vi "stimulate_and_record_async_daq_temp.vi"(3 "SSH password":string, 4 "Transfer and Run Date Folder After Experiment":bool, 5 "SSH user name":string, 6 "Tags":string, 7 "Frames":i32, 8 "Convert Power to Voltage":bool, 9 "voltages/power":dbl[](array[numeric]), 10 "parameters":string[](array[string]), 11 "parameters headers":string[](array[string])) -> ()   [LabVIEW 2016]
uses:
  <vilib>/vision/driver/IMAQdx.llb/IMAQdx Acquisition Mode.ctl
  <vilib>/userdefined/High Color/IMAQdx.ctl
  <vilib>/vision/driver/IMAQdx.llb/IMAQdx Buffer Number Mode.ctl
  <vilib>/Utility/file.llb/Write To Spreadsheet File (DBL).vi
  <vilib>/Utility/file.llb/Write To Spreadsheet File (string).vi
  <vilib>/Utility/file.llb/Read From Spreadsheet File (string).vi
  <vilib>/vision/driver/NI_Vision_Acquisition_Software.lvlib
panel:
  out "DAC0 Voltage":dbl format="%.6f"
  out "Saved Buffer Number":u32
  out "ProcessFrameRate":dbl
  out "# elements in queue":i32
  out "CameraFrameRate":dbl
  out "Camera Buffer Number":u32
  out "Image":T1(plugin-control)
  out "JPEG Quality":dbl
  out "Save Directory":path
  in  "stop":bool
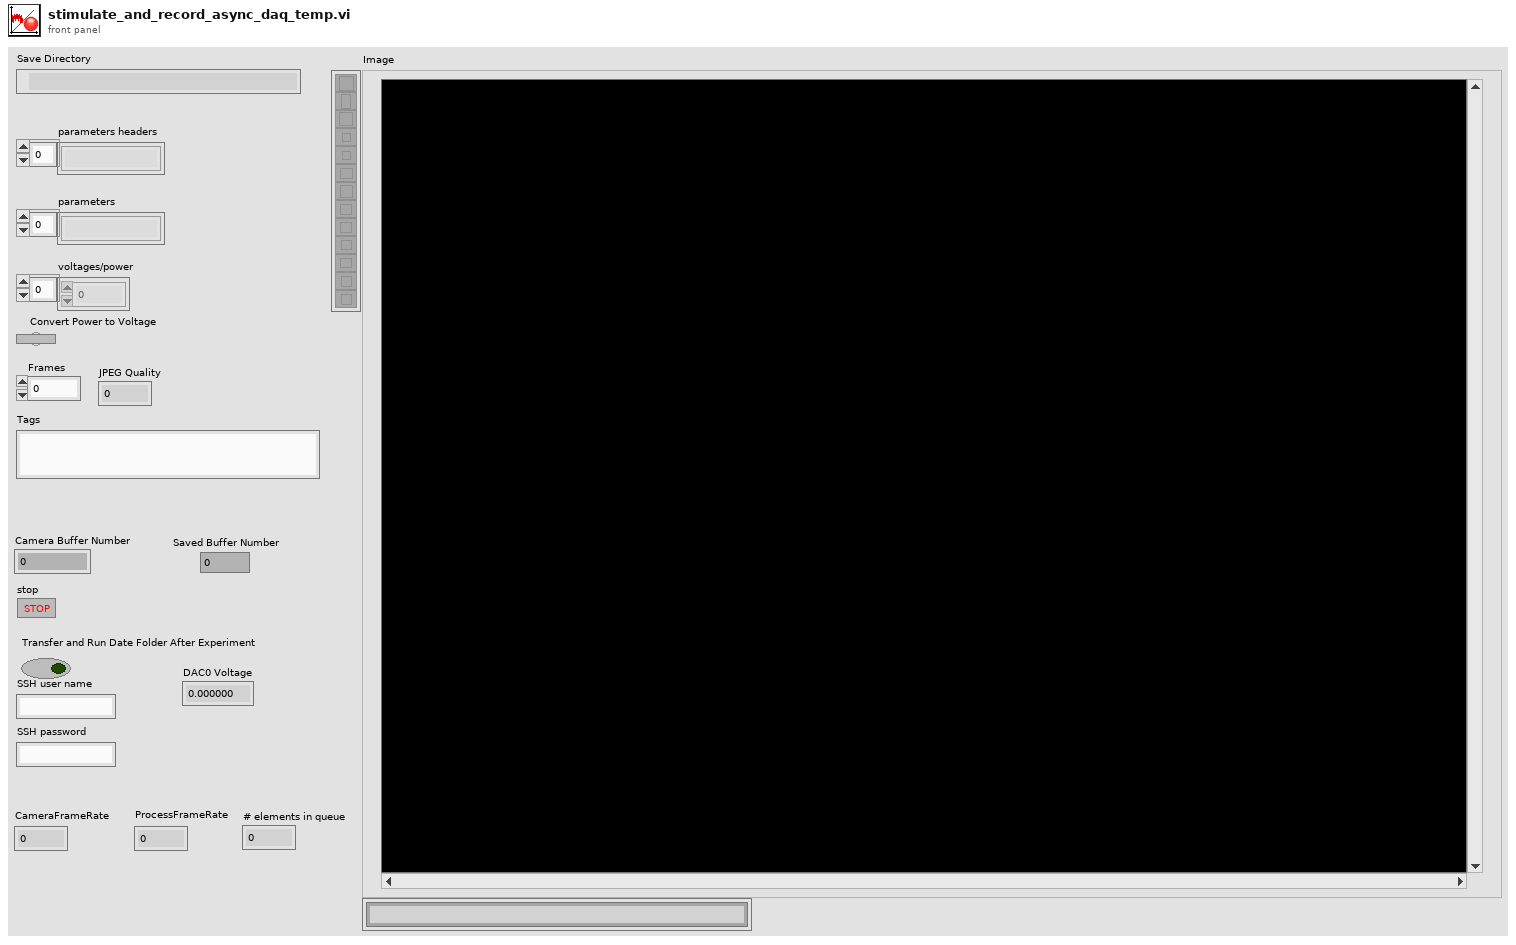
[diagram p1: front panel]
types:
  T1 = typedef "IMAQ Image.ctl" = refnum<image>
  T2 = typedef "IMAQdx.ctl" = refnum<k21>
  T3 = typedef "NI_Vision_Acquisition_Software.lvlib/IMAQdx Buffer Number Mode.ctl" = enum32{"Next", "Last", "Buffer Number", "Every", "Last New"}
  T4 = typedef "Image Type" = u32
  T5 = typedef "NI_Vision_Acquisition_Software.lvlib/IMAQdx Acquisition Mode.ctl" = enum32{"One Shot", "Continuous"}
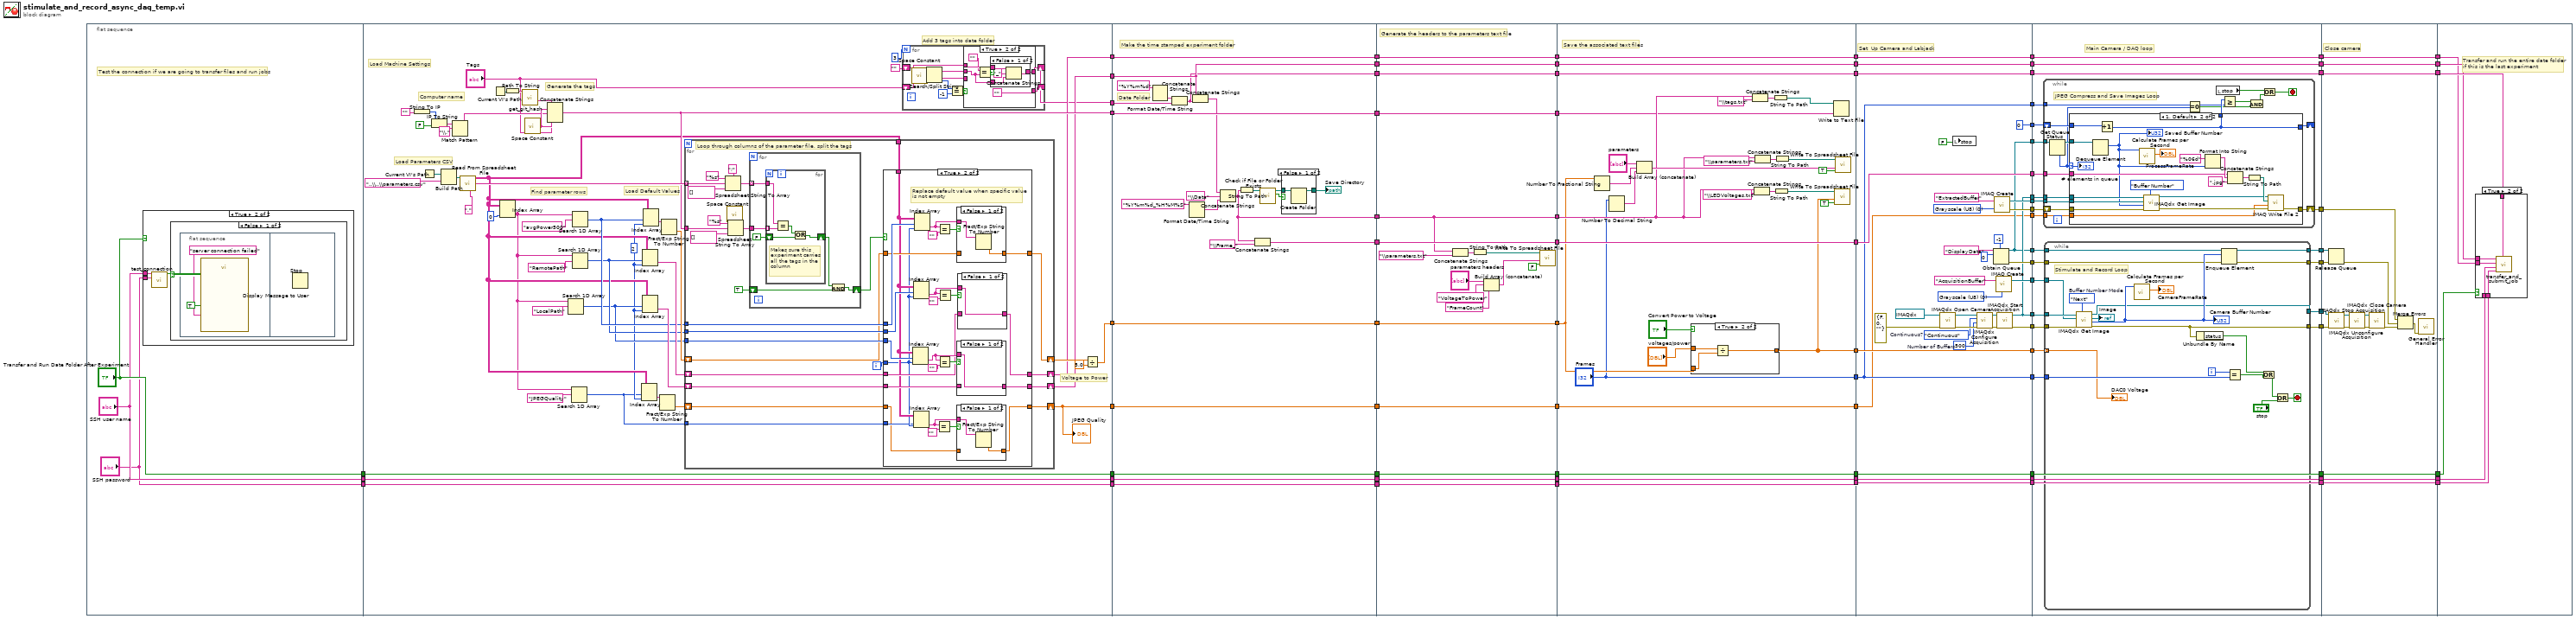
[diagram p0: block diagram]
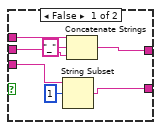
[diagram p4: hidden frame]
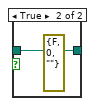
[diagram p11: hidden frame]
diagram:
  n1 = flat-sequence {
    tunnel: ["Transfer and Run Date Folder After Experiment"] -> w47
    tunnel: ["SSH user name"] -> w46
    tunnel: ["SSH password"] -> w45
    tunnel: [w129] -> w77
    tunnel: [w112] -> w76
    tunnel: [w103] -> w67
    tunnel: [w104] -> w66
    tunnel: w47 -> [w121]
    tunnel: w46 -> [w120]
    tunnel: w45 -> [w119]
    tunnel: [w121] -> w38
    tunnel: [w120] -> w31
    tunnel: [w119] -> w30
    tunnel: [w100] -> w23
    tunnel: [w91] -> w22
    tunnel: [w265] -> w61
    tunnel: [w264] -> w59
    tunnel: [w263] -> w57
    tunnel: [w262] -> w55
    tunnel: [w244] -> w53
    tunnel: [w246] -> w51
    tunnel: [w261] -> w49
    tunnel: w66 -> [w261]
    tunnel: w67 -> [w246]
    tunnel: w76 -> [w262]
    tunnel: w77 -> [w263]
    tunnel: [w253] -> w39
    tunnel: w38 -> [w253]
    tunnel: [w252] -> w32
    tunnel: w31 -> [w252]
    tunnel: w30 -> [w251]
    tunnel: [w251] -> w29
    tunnel: w23 -> [w247]
    tunnel: w22 -> [w243]
    tunnel: [w243] -> w19
    tunnel: w61 -> [w287]
    tunnel: [w287] -> w60
    tunnel: w59 -> [w273]
    tunnel: [w273] -> w58
    tunnel: w57 -> [w286]
    tunnel: [w286] -> w56
    tunnel: w55 -> [w285]
    tunnel: [w285] -> w54
    tunnel: w53 -> [w284]
    tunnel: [w284] -> w52
    tunnel: w51 -> [w283]
    tunnel: [w283] -> w50
    tunnel: w49 -> [w282]
    tunnel: [w282] -> w48
    tunnel: [w272] -> w40
    tunnel: w39 -> [w272]
    tunnel: [w271] -> w33
    tunnel: w32 -> [w271]
    tunnel: w29 -> [w270]
    tunnel: [w270] -> w28
    tunnel: [w269] -> w20
    tunnel: w19 -> [w269]
    tunnel: w60 -> [w315]
    tunnel: [w315] -> w82
    tunnel: [w298] -> w80
    tunnel: ["Frames"] -> w79
    tunnel: w58 -> [w307]
    tunnel: w56 -> [w294]
    tunnel: w54 -> [w289]
    tunnel: w52 -> [w303]
    tunnel: [w303] -> w72
    tunnel: [w302] -> w68
    tunnel: w50 -> [w302]
    tunnel: [w301] -> w62
    tunnel: w48 -> [w301]
    tunnel: [w292] -> w41
    tunnel: w40 -> [w292]
    tunnel: [w291] -> w34
    tunnel: w33 -> [w291]
    tunnel: w28 -> [w290]
    tunnel: [w290] -> w27
    tunnel: [w288] -> w21
    tunnel: w20 -> [w288]
    tunnel: w82 -> [w327]
    tunnel: [w355] -> w81
    tunnel: w80 -> [w355]
    tunnel: w79 -> [w326]
    tunnel: [w326] -> w78
    tunnel: [w354] -> w73
    tunnel: w72 -> [w354]
    tunnel: [w353] -> w69
    tunnel: w68 -> [w353]
    tunnel: [w352] -> w63
    tunnel: w62 -> [w352]
    tunnel: [w351] -> w42
    tunnel: w41 -> [w351]
    tunnel: [w350] -> w35
    tunnel: w34 -> [w350]
    tunnel: w27 -> [w349]
    tunnel: [w349] -> w26
    tunnel: w21 -> [w324]
    tunnel: [w333] -> w18
    tunnel: [w328] -> w17
    tunnel: [w332] -> w16
    tunnel: [w331] -> w15
    tunnel: [w325] -> w14
    tunnel: [w330] -> w11
    tunnel: [w329] -> w10
    tunnel: [w328] -> w9
    tunnel: [w327] -> w8
    tunnel: [w326] -> w7
    tunnel: [w325] -> w6
    tunnel: [w324] -> w5
    tunnel: [0] -> w2
    tunnel: w81 -> [w381]
    tunnel: w78 -> [w380]
    tunnel: [w379] -> w74
    tunnel: w73 -> [w379]
    tunnel: [w378] -> w70
    tunnel: w69 -> [w378]
    tunnel: [w377] -> w64
    tunnel: w63 -> [w377]
    tunnel: [w376] -> w43
    tunnel: w42 -> [w376]
    tunnel: [w375] -> w36
    tunnel: w35 -> [w375]
    tunnel: w26 -> [w374]
    tunnel: [w374] -> w25
    tunnel: w18 -> [w373]
    tunnel: w17 -> [w372]
    tunnel: w16 -> [w371]
    tunnel: w15 -> [w370]
    tunnel: w14 -> [w369]
    tunnel: [w368] -> w13
    tunnel: [w367] -> w12
    tunnel: w11 -> [w366]
    tunnel: w10 -> [w365]
    tunnel: w9 -> [w364]
    tunnel: w8 -> [w363]
    tunnel: w7 -> [w362]
    tunnel: w6 -> [w361]
    tunnel: w5 -> [w360]
    tunnel: [w357] -> w4
    tunnel: [w359] -> w3
    tunnel: w2 -> [w358]
    tunnel: [w356] -> w1
    tunnel: [w459] -> w75
    tunnel: w74 -> [w459]
    tunnel: [w458] -> w71
    tunnel: w70 -> [w458]
    tunnel: [w457] -> w65
    tunnel: w64 -> [w457]
    tunnel: [w456] -> w44
    tunnel: w43 -> [w456]
    tunnel: [w455] -> w37
    tunnel: w36 -> [w455]
    tunnel: w25 -> [w454]
    tunnel: [w454] -> w24
    tunnel: w13 -> [w449]
    tunnel: w12 -> [w448]
    tunnel: w4 -> [w445]
    tunnel: w3 -> [w444]
    tunnel: w1 -> [w443]
    tunnel: w75 -> [w465]
    tunnel: w71 -> [w464]
    tunnel: w65 -> [w463]
    tunnel: w44 -> [w462]
    tunnel: w37 -> [w461]
    tunnel: w24 -> [w460]
    frame #0 {
      # "Test the connection if we are going to transfer files and run jobs"
      n2 = case shown="True" "Transfer and Run Date Folder After Experiment" {
        tunnel: "SSH password" -> [_ w88]
        tunnel: "SSH user name" -> [_ w86]
        frame False {
        }
        frame True {
          n3 = call "test_connection.vi"("Username"=w86, "Password"=w88) -> ("Connection Successful"=w87:bool)  [unwired: 7 in]
          n4 = case shown="False" w87 {
            frame False {
              n5 = flat-sequence {
                frame #0 {
                  n6 = call "Display Message to User"("Enable"=TRUE, "Message"="server connection failed") -> ()  [unwired: 8 in, 2 out]
                }
                frame #1 {
                  n7 = Stop() -> ()  [unwired: 1 in]
                }
              }
            }
            frame True {
            }
          }
        }
      }
    }
    frame #1 {
      w94 = 2
      # "Add 3 tags into date folder"
      # "Generate the tags"
      # "Find parameter rows"
      # "Load Default Values"
      # "Voltage to Power"
      # "Load Parameters CSV"
      # "Computer name"
      # "Load Machine Settings"
      n8 = String To IP(1:"") -> (0:w137:u32)
      n9 = Current VI's Path() -> (path=w132:path)
      n10 = IP To String(1:FALSE, 2:w137) -> (0:w134:string)
      n11 = Build Path(base path=w132, name or relative path="..\\..\\parameters.csv") -> (appended path=w123:path)
      n12 = Match Pattern(string=w134, regular expression="\\.") -> (before substring=w114:string)  [unwired: 1 in, 3 out]
      n13 = call-poly <vilib>:"Read From Spreadsheet File.vi"("delimiter (\\t)"=",", "file path (dialog if empty)"=w123) -> ("first row"=w113:string[], "all rows"=w96:string[][])  [unwired: 5 in, 3 out]
      n14 = Current VI's Path() -> (path=w116:path)
      n15 = Index Array(array=w96, index (col)=0) -> (element=w95:string[])  [unwired: 1 in]
      n16 = Path To String(path=w116) -> (string=w115:string)
      n17 = call "get_git_hash.vi"("VI folder"=w115) -> ("github hash"=w118:string)  [unwired: 10 in]
      n18 = call <vilib>:"Space Constant.vi"() -> ("String"=w117:string)
      n19 = Concatenate Strings(w118, w117, w114, w117, "Tags") -> (w112:string)
      n20 = Search 1D Array(1D array=w95, element="LocalPath") -> (index of element=w106:i32)  [unwired: 1 in]
      n21 = Search 1D Array(1D array=w95, element="JPEGQuality") -> (index of element=w92:i32)  [unwired: 1 in]
      n22 = Search 1D Array(1D array=w95, element="RemotePath") -> (index of element=w107:i32)  [unwired: 1 in]
      n23 = Search 1D Array(1D array=w95, element="avgPower500") -> (index of element=w108:i32)  [unwired: 1 in]
      n24 = Index Array(array=w96, index (row)=w92, index (col)=w94) -> (element=w97:string)
      n25 = Index Array(array=w96, index (row)=w107, index (col)=w94) -> (element=w110:string)
      n26 = Index Array(array=w96, index (row)=w106, index (col)=w94) -> (element=w109:string)
      n27 = Index Array(array=w96, index (row)=w108, index (col)=w94) -> (element=w125:string)
      n28 = Fract/Exp String To Number(string=w97) -> (number=w93:dbl)  [unwired: 3 in, 1 out]
      n29 = Fract/Exp String To Number(string=w125) -> (number=w111:dbl)  [unwired: 3 in, 1 out]
      n30 = for {
        tunnel: w113 -> [w191] mode=indexing
        tunnel: w112 -> [w183]
        tunnel: w108 -> [w178]
        tunnel: w107 -> [w177]
        tunnel: w106 -> [w176]
        tunnel: w96 -> [w181]
        shift-right: [w173] -> w105
        shift-left: w111 -> [w174]
        shift-right: [w170] -> w104
        shift-left: w110 -> [w171]
        shift-right: [w169] -> w103
        shift-left: w109 -> [w172]
        shift-right: [w166] -> w91
        shift-left: w93 -> [w168]
        tunnel: w92 -> [w167]
        i -> [w175]
        # "Loop through columns of the parameter file, split the tags"
        n31 = Spreadsheet String To Array(delimiter (Tab)=";", format string="%s", spreadsheet string=w191, array type (2D Dbl)=string[] []) -> (array=w187:string[])
        n32 = call <vilib>:"Space Constant.vi"() -> ("String"=w185:string)
        n33 = Spreadsheet String To Array(delimiter (Tab)=w185, format string="%s", spreadsheet string=w183, array type (2D Dbl)=string[] []) -> (array=w182:string[])
        n34 = for {
          tunnel: w187 -> [w237] mode=indexing
          tunnel: w182 -> [w236]
          shift-right: [w234] -> w179
          shift-left: TRUE -> [w232]
          n35 = for {
            tunnel: w237 -> [w242]
            tunnel: w236 -> [w241] mode=indexing
            shift-right: [w238] -> w233
            shift-left: FALSE -> [w239]
            # "Makes sure this\nexperiment carries\nall the tags in the\ncolumn"
            n36 = Equal?(x=w242, y=w241) -> (x = y?=w240:bool)
            n37 = Or(x=w240, y=w239) -> (x .or. y?=w238:bool)
          }
          n38 = And(x=w233, y=w232) -> (x .and. y?=w234:bool)
        }
        n39 = case shown="True" w179 {
          tunnel: w174 -> [w195 w216]
          tunnel: [w195 w215] -> w173
          tunnel: w178 -> [_ w221]
          tunnel: w177 -> [_ w220]
          tunnel: w176 -> [_ w219]
          tunnel: w175 -> [_ w198]
          tunnel: w181 -> [_ w199]
          tunnel: [w194 w205] -> w170
          tunnel: [w193 w207] -> w169
          tunnel: w172 -> [w193 w206]
          tunnel: w171 -> [w194 w204]
          tunnel: w168 -> [w192 w196]
          tunnel: w167 -> [_ w197]
          tunnel: [w192 w200] -> w166
          frame False {
          }
          frame True {
            # "Replace default value when specific value\nis not empty"
            n40 = Index Array(array=w199, index (row)=w219, index (col)=w198) -> (element=w208:string)
            n41 = Index Array(array=w199, index (row)=w220, index (col)=w198) -> (element=w211:string)
            n42 = Index Array(array=w199, index (row)=w197, index (col)=w198) -> (element=w201:string)
            n43 = Index Array(array=w199, index (row)=w221, index (col)=w198) -> (element=w214:string)
            n44 = Equal?(x=w201, y="") -> (x = y?=w202:bool)
            n45 = Equal?(x=w214, y="") -> (x = y?=w217:bool)
            n46 = Equal?(x=w208, y="") -> (x = y?=w209:bool)
            n47 = Equal?(x=w211, y="") -> (x = y?=w212:bool)
            n48 = case shown="False" w202 {
              tunnel: w196 -> [_ w224]
              tunnel: [w223 w224] -> w200
              tunnel: w201 -> [w222 _]
              frame False {
                n49 = Fract/Exp String To Number(string=w222) -> (number=w223:dbl)  [unwired: 3 in, 1 out]
              }
              frame True {
              }
            }
            n50 = case shown="False" w217 {
              tunnel: w216 -> [_ w231]
              tunnel: [w230 w231] -> w215
              tunnel: w214 -> [w229 _]
              frame False {
                n51 = Fract/Exp String To Number(string=w229) -> (number=w230:dbl)  [unwired: 3 in, 1 out]
              }
              frame True {
              }
            }
            n52 = case shown="False" w209 {
              tunnel: w208 -> [w225 _]
              tunnel: [w225 w226] -> w207
              tunnel: w206 -> [_ w226]
              frame False {
              }
              frame True {
              }
            }
            n53 = case shown="False" w212 {
              tunnel: w211 -> [w227 _]
              tunnel: [w227 w228] -> w205
              tunnel: w204 -> [_ w228]
              frame False {
              }
              frame True {
              }
            }
          }
        }
      }
      "JPEG Quality" <- w91
      n54 = for {
        N: 3 -> [_]
        shift-right: [w138] -> _
        shift-left: "Tags" -> [w147]
        shift-right: [w140] -> w100
        shift-left: "" -> [w145]
        n55 = call <vilib>:"Space Constant.vi"() -> ("String"=w146:string)
        n56 = Search/Split String(string=w147, search string/char (-)=w146) -> (substring before match=w144:string, match + rest of string=w143:string, offset of match=w142:i32)  [unwired: 1 in]
        n57 = Equal?(x=w142, y=-1) -> (x = y?=w139:bool)
        n58 = case shown="True" w139 {
          tunnel: w145 -> [w148 w158]
          tunnel: w144 -> [w149 w155]
          tunnel: w143 -> [w150 _]
          tunnel: [w152 ""] -> w138
          tunnel: [w151 w157] -> w140
          frame False {
            n59 = String Subset(string=w150, offset (0)=1) -> (substring=w152:string)  [unwired: 1 in]
            n60 = Concatenate Strings(w148, "_", w149) -> (w151:string)
          }
          frame True {
            n61 = Equal?(x="", y=w155) -> (x = y?=w159:bool)
            n62 = case shown="False" w159 {
              tunnel: w158 -> [w162 w165]
              tunnel: [w163 w165] -> w157
              tunnel: w155 -> [w161 _]
              frame False {
                n63 = Concatenate Strings(w162, "_", w161) -> (w163:string)
              }
              frame True {
              }
            }
          }
        }
      }
      n64 = Divide(x=w105, y=5.0) -> (x/y=w129:dbl)
    }
    frame #2 {
      # "Make the time stamped experiment folder"
      # "Date Folder"
      n65 = Format Date/Time String(time format string (%c)="%Y%m%d") -> (date/time string=w248:string)  [unwired: 2 in]
      n66 = Concatenate Strings(w248, w247) -> (w244:string)
      n67 = Format Date/Time String(time format string (%c)="%Y%m%d_%H%M%S") -> (date/time string=w250:string)  [unwired: 2 in]
      n68 = Concatenate Strings(w246, w244) -> (w245:string)
      n69 = Concatenate Strings(w245, "\\Data", w250) -> (w264:string)
      n70 = String To Path(string=w264) -> (path=w256:path)
      n71 = Concatenate Strings(w264, "\\Frame_") -> (w265:string)
      n72 = call <vilib>:"Check if File or Folder Exists.vi"("path"=w256) -> ("file or folder exists?"=w259:bool, "dup path"=w258:path)  [unwired: 8 in, 1 out]
      n73 = case shown="False" w259 {
        tunnel: [w266 w268] -> w255
        tunnel: w258 -> [w267 w268]
        frame False {
          n74 = Create Folder(path (use dialog)=w267) -> (created path=w266:path)  [unwired: 2 in, 2 out]
        }
        frame True {
          (unwired) errorcluster {"status"=FALSE, "code"=0, "source"=""} ("error out")
        }
      }
      "Save Directory" <- w255
    }
    frame #3 {
      # "Generate the headers to the parameters text file"
      n75 = Concatenate Strings(w273, "\\parameters.txt") -> (w281:string)
      n76 = String To Path(string=w281) -> (path=w280:path)
      n77 = Build Array (concatenate)("parameters headers", "VoltageToPower", "FrameCount") -> (w277:string[])
      n78 = call-poly <vilib>:"Write To Spreadsheet File.vi"("append to file? (new file:F)"=FALSE, "1D data"=w277, "file path (dialog if empty)"=w280) -> ()  [unwired: 5 in, 1 out]
    }
    frame #4 {
      # "Save the associated text files"
      n79 = Number To Fractional String(number=w294) -> (F-format string=w295:string)  [unwired: 3 in]
      n80 = Number To Decimal String(number="Frames") -> (decimal integer string=w296:string)  [unwired: 1 in]
      n81 = Build Array (concatenate)("parameters", w295, w296) -> (w308:string[])
      n82 = case shown="True" "Convert Power to Voltage" {
        tunnel: "voltages/power" -> [w318 w321]
        tunnel: [w318 w319] -> w298
        tunnel: w294 -> [_ w320]
        frame False {
        }
        frame True {
          n83 = Divide(x=w321, y=w320) -> (x/y=w319:dbl[])
        }
      }
      n84 = Concatenate Strings(w307, "\\tags.txt") -> (w305:string)
      n85 = Concatenate Strings(w307, "\\LEDVoltages.txt") -> (w317:string)
      n86 = Concatenate Strings(w307, "\\parameters.txt") -> (w312:string)
      n87 = String To Path(string=w305) -> (path=w304:path)
      n88 = String To Path(string=w317) -> (path=w316:path)
      n89 = String To Path(string=w312) -> (path=w311:path)
      n90 = Write to Text File(file (use dialog)=w304, text=w289) -> ()  [unwired: 2 in, 3 out]
      n91 = call-poly <vilib>:"Write To Spreadsheet File.vi"("append to file? (new file:F)"=TRUE, "1D data"=w298, "file path (dialog if empty)"=w316) -> ()  [unwired: 5 in, 1 out]
      n92 = call-poly <vilib>:"Write To Spreadsheet File.vi"("append to file? (new file:F)"=TRUE, "1D data"=w308, "file path (dialog if empty)"=w311) -> ()  [unwired: 5 in, 1 out]
    }
    frame #5 {
      w336 = T4 0 items=["Grayscale (U8)", "Grayscale (I16)", "Grayscale (SGL)", "Complex (CSG)", "RGB (U32)", "HSL (U32)", "RGB (U64)"] ("Image Type")
      w345 = T4 0 items=["Grayscale (U8)", "Grayscale (I16)", "Grayscale (SGL)", "Complex (CSG)", "RGB (U32)", "HSL (U32)", "RGB (U64)"] ("Image Type")
      w346 = u32 500  # Number of Buffers
      w342 = IMAQdx_Acquisition_Mode."Continuous"  # Continuous?
      # "Set  Up Camera and Labjack"
      n93 = call <vilib>:"IMAQdx Open Camera.vi"("error in"=errorcluster {"status"=FALSE, "code"=0, "source"=""}, "Session In"=T2 "cam0") -> ("error out"=w347:errorcluster, "Session Out"=w348:T2)  [unwired: 8 in]
      n94 = local write "stop"(FALSE) -> ()
      n95 = call <vilib>:"IMAQdx Configure Acquisition.vi"("error in"=w347, "Number of Buffers"=w346, "Continuous?"=w342, "Session In"=w348) -> ("error out"=w343:errorcluster, "Session Out"=w341:T2)  [unwired: 6 in]
      n96 = Obtain Queue(max queue size (-1, unlimited)=-1, name (unnamed)="DisplayData", element data type=u32 0) -> (queue out=w325:refnum<queue>, error out=w331:errorcluster)  [unwired: 2 in, 1 out]
      n97 = call "IMAQ Create"("Image Name"="ExtractedBuffer", "Image Type"=w336) -> ("New Image"=w329:T1, "error out"=w330:errorcluster)  [unwired: 3 in]
      n98 = call "IMAQ Create"("Image Name"="AcquisitionBuffer", "Image Type"=w345) -> ("New Image"=w332:T1)  [unwired: 3 in, 1 out]
      n99 = call <vilib>:"IMAQdx Start Acquisition.vi"("error in"=w343, "Session In"=w341) -> ("error out"=w333:errorcluster, "Session Out"=w328:T2)  [unwired: 8 in]
    }
    frame #6 {
      # "Main Camera / DAQ loop"
      n100 = while {
        tunnel: w361 -> [w399]
        tunnel: w365 -> [w397]
        tunnel: w364 -> [w396]
        tunnel: w363 -> [w394]
        shift-right: [w393] -> w359
        shift-left: w366 -> [w395]
        tunnel: w362 -> [w386]
        tunnel: w360 -> [w391]
        shift-right: [w388] -> _
        shift-left: w358 -> [w389]
        stop <- w392 stop-if-true
        # "JPEG Compress and Save Images Loop"
        n101 = Get Queue Status(queue=w399) -> (queue out=w398:refnum<queue>, # elements in queue=w382:i32)  [unwired: 2 in, 6 out]
        n102 = case shown="1, Default" w382 {
          selector: w382 -> [_ w420]
          tunnel: w398 -> [_ w418]
          tunnel: w397 -> [_ w417]
          tunnel: w396 -> [_ w416]
          tunnel: w395 -> [w401 w415]
          tunnel: w394 -> [_ w409]
          tunnel: [w401 w405] -> w393
          tunnel: w391 -> [_ w404]
          tunnel: w389 -> [w400 w403]
          tunnel: [w400 w402] -> w388
          tunnel: [w400 w402] -> w387
          frame 0 {
          }
          frame 1, Default {
            n103 = Dequeue Element(queue=w418) -> (element=w406:u32)  [unwired: 2 in, 3 out]
            "Saved Buffer Number" <- w406
            n104 = Increment(x=w403) -> (x+1=w402:i32)
            n105 = call <vilib>:"Calculate Frames per Second.vi"("Buffer Number"=w406) -> ("Processed Frames/s"=→"ProcessFrameRate":dbl)  [unwired: 8 in, 2 out]
            n106 = call <vilib>:"IMAQdx Get Image.vi"("Buffer Number Mode (Next)"=IMAQdx_Buffer_Number_Mode."Buffer Number", "error in"=w415, "Buffer Number In"=w406, "Image In"=w417, "Session In"=w416) -> ("error out"=w407:errorcluster, "Image Out"=w408:T1)  [unwired: 3 in, 2 out]
            n107 = Format Into String(format string="%06d" ("string"), w406) -> (resulting string=w411:string)  [unwired: 2 in, 1 out]
            n108 = Concatenate Strings(w409, w411, ".jpg" ("string")) -> (w413:string)
            n109 = String To Path(string=w413) -> (path=w412:path)
            n110 = call-poly "IMAQ Write File 2"("error in (no error)"=w407, "Image Quality"=w404, "File Path"=w412, "Image"=w408) -> ("error out"=w405:errorcluster)  [unwired: 6 in, 1 out]
            "# elements in queue" <- w420
          }
        }
        n111 = Equal To 0?(x=w382) -> (x = 0?=w383:bool)
        n112 = local read "stop"() -> (w390:bool)
        n113 = Greater Or Equal?(x=w387, y=w386) -> (x >= y?=w385:bool)
        n114 = And(x=w385, y=w383) -> (x .and. y?=w384:bool)
        n115 = Or(x=w390, y=w384) -> (x .or. y?=w392:bool)
      }
      n116 = while {
        tunnel: w381 -> [w422] mode=indexing
        tunnel: w380 -> [w439]
        tunnel: w373 -> [w434]
        tunnel: w372 -> [w433]
        tunnel: w371 -> [w432]
        tunnel: w370 -> [w431]
        tunnel: w369 -> [w430]
        tunnel: [w427] -> w356
        tunnel: [w426] -> w357
        tunnel: [w425] -> w368
        tunnel: [w424] -> w367
        i -> [w440]
        stop <- w442 stop-if-true
        w438 = IMAQdx_Buffer_Number_Mode."Next"  # Buffer Number Mode
        # "Stimulate and Record Loop"
        n117 = call <vilib>:"IMAQdx Get Image.vi"("Buffer Number Mode (Next)"=w438, "error in"=w434, "Image In"=w432, "Session In"=w433) -> ("error out"=w424:errorcluster, "Buffer Number Out"=w435:u32, "Image Out"=→"Image":T1, "Session Out"=w425:T2)  [unwired: 4 in]
        "Camera Buffer Number" <- w435
        n118 = call <vilib>:"Calculate Frames per Second.vi"("Buffer Number"=w435) -> ("Processed Frames/s"=→"CameraFrameRate":dbl)  [unwired: 8 in, 2 out]
        n119 = Unbundle By Name(w424) -> ("status"=w429:bool)
        n120 = Enqueue Element(queue=w430, element=w435, error in (no error)=w431) -> (queue out=w427:refnum<queue>, error out=w426:errorcluster)  [unwired: 1 in, 1 out]
        n121 = Equal?(x=w440, y=w439) -> (x = y?=w423:bool)
        n122 = Or(x=w429, y=w423) -> (x .or. y?=w428:bool)
        n123 = Or(x=w428, y="stop") -> (x .or. y?=w442:bool)
        "DAC0 Voltage" <- w422
      }
    }
    frame #7 {
      # "Close camera"
      n124 = Release Queue(queue=w443) -> ()  [unwired: 2 in, 3 out]
      n125 = call <vilib>:"IMAQdx Stop Acquisition.vi"("error in"=w448, "Session In"=w449) -> ("error out"=w450:errorcluster, "Session Out"=w451:T2)  [unwired: 8 in]
      n126 = call <vilib>:"IMAQdx Unconfigure Acquisition.vi"("error in"=w450, "Session In"=w451) -> ("error out"=w453:errorcluster, "Session Out"=w452:T2)  [unwired: 8 in]
      n127 = call <vilib>:"IMAQdx Close Camera.vi"("error in"=w453, "Session In"=w452) -> ("error out"=w446:errorcluster)  [unwired: 9 in]
      n128 = Merge Errors(w444, w445, w446) -> (w447:errorcluster)
      n129 = call <vilib>:"General Error Handler.vi"("error in (no error)"=w447) -> ()  [unwired: 10 in, 5 out]
    }
    frame #8 {
      # "Transfer and run the entire date folder\nif this is the last experiment"
      n130 = case shown="True" w462 {
        tunnel: w465 -> [_ w470]
        tunnel: w464 -> [_ w469]
        tunnel: w463 -> [_ w468]
        tunnel: w461 -> [_ w467]
        tunnel: w460 -> [_ w466]
        frame False {
        }
        frame True {
          n131 = call "transfer_and_submit_job.vi"("Date Folder"=w470, "Password"=w466, "Username"=w467, "Remote Data Directory"=w468, "Local Data Directory"=w469) -> ()  [unwired: 7 in]
        }
      }
    }
  }
